vi "apply tracking setting.vi"(7 "tracking?":bool, 9 "tracking settings":T3, 10 "tracking state in":T1) -> (2 "tracking state out":T1={"x state"={"pos estimate"=0.0, "v estimate"=0.0, "weighted position error sum"=0.0, "photon count"=0, "transmit tick count"=0, "axis number"=0, "px (levels^2)"=0.0, "pxv (levels^2/ticks)"=0.0, "pv (levels^2/ticks^2)"=0.0, "vel diff (levels^2/ticks^3)"=0.0, "gx"=0.0, "rtwiddle"=0.0, "photon count ch0"=0, "photon count ch1"=0, "Dx -levels^2/ticks"=0.0}, "y state"={"pos estimate"=0.0, "v estimate"=0.0, "weighted position error sum"=0.0, "photon count"=0, "transmit tick count"=0, "axis number"=1, "px (levels^2)"=0.0, "pxv (levels^2/ticks)"=0.0, "pv (levels^2/ticks^2)"=0.0, "vel diff (levels^2/ticks^3)"=0.0, "gx"=0.0, "rtwiddle"=0.0, "photon count ch0"=0, "photon count ch1"=0, "Dx -levels^2/ticks"=0.0}, "z state"={"pos estimate"=0.0, "v estimate"=0.0, "weighted position error sum"=0.0, "photon count"=0, "transmit tick count"=0, "axis number"=2, "px (levels^2)"=0.0, "pxv (levels^2/ticks)"=0.0, "pv (levels^2/ticks^2)"=0.0, "vel diff (levels^2/ticks^3)"=0.0, "gx"=0.0, "rtwiddle"=0.0, "photon count ch0"=0, "photon count ch1"=0, "Dx -levels^2/ticks"=0.0}, "spot number"=0})   [LabVIEW 2010]
uses:
  polar tracking settings.ctl
  kalman 3-axis state.ctl
  integrating single axis kalman state.ctl
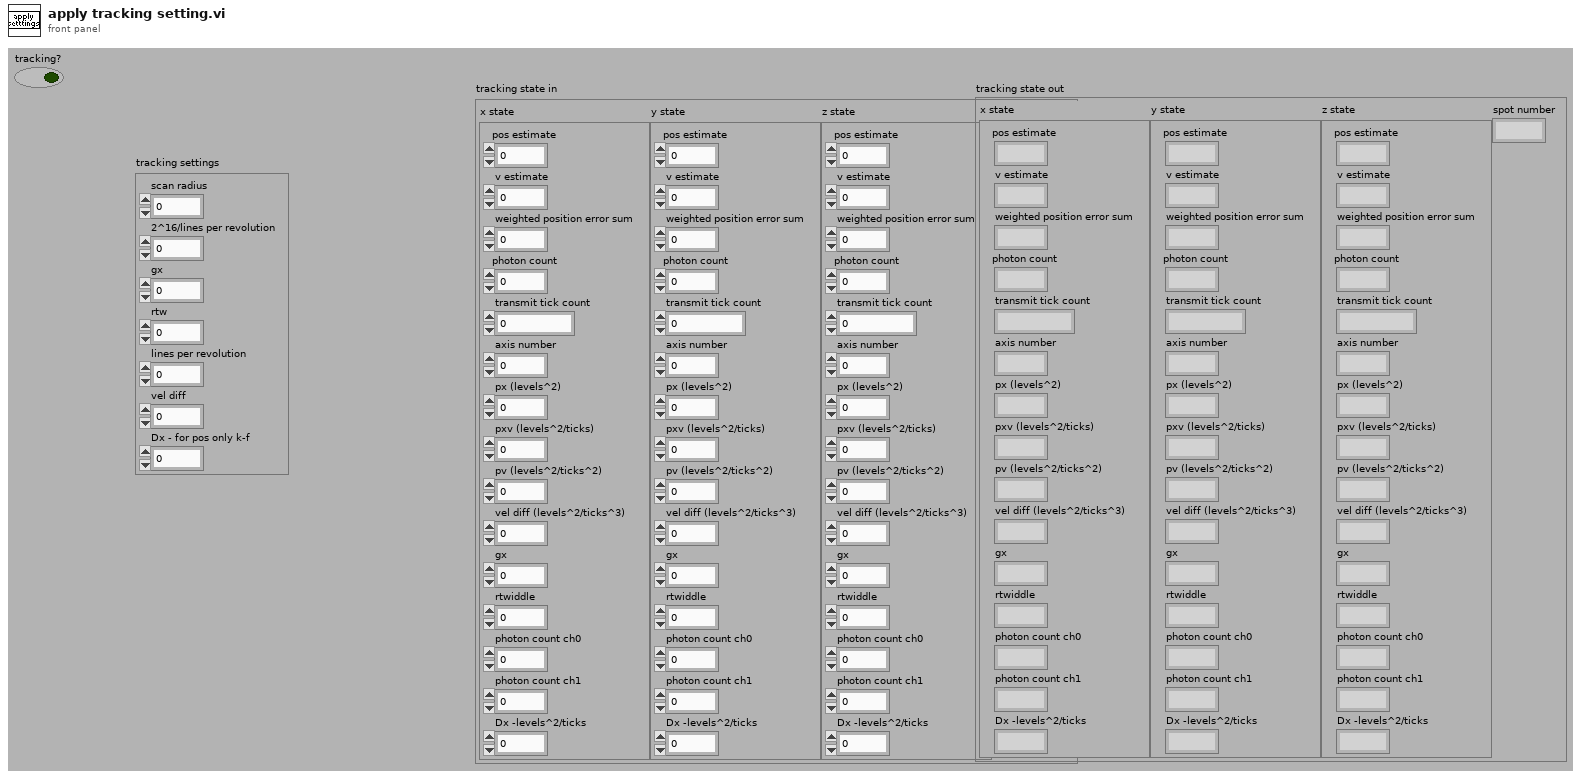
[diagram p1: front panel]
types:
  T1 = typedef "kalman 3-axis state.ctl" = cluster{"x state":T2, "y state":T2, "z state":T2, "spot number":u8}
  T2 = typedef "integrating single axis kalman state.ctl" = cluster{"pos estimate":fxp<+/-,32,16>, "v estimate":fxp<+/-,16,0>, "weighted position error sum":fxp<+/-,32,32>, "photon count":u32, "transmit tick count":u32, "axis number":u8, "px (levels^2)":fxp<+,32,19>, "pxv (levels^2/ticks)":fxp<+,32,2>, "pv (levels^2/ticks^2)":fxp<+,32,-14>, "vel diff (levels^2/ticks^3)":fxp<+,24,-22>, "gx":fxp<+,16,8>, "rtwiddle":fxp<+,16,26>, "photon count ch0":u32, "photon count ch1":u32, "Dx -levels^2/ticks":fxp<+,32,19>}
  T3 = typedef "polar tracking settings.ctl" = cluster{"scan radius":u16, "2^16/lines per revolution":u16, "gx":fxp<+,16,8>, "rtw":fxp<+,16,26>, "lines per revolution":u8, "vel diff":fxp<+,24,-22>, "Dx - for pos only k-f":fxp<+,32,19>}
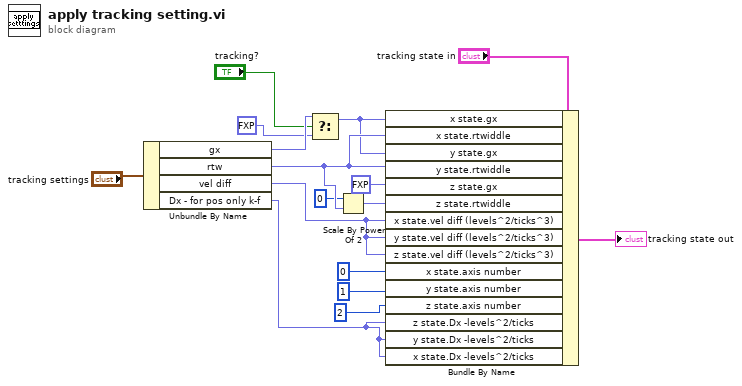
[diagram p0: block diagram]
diagram:
  n1 = Unbundle By Name("tracking settings") -> ("gx"=w3:fxp<+,16,8>, "rtw"=w13:fxp<+,16,26>, "vel diff"=w10:fxp<+,24,-22>, "Dx - for pos only k-f"=w6:fxp<+,32,19>)
  n2 = Select(t=w3, s="tracking?", f=fxp<+,16,8> 1.0) -> (s? t:f=w4:fxp<+,16,8>)
  n3 = Scale By Power Of 2(n=0, x=w13) -> (x*2^n=w11:fxp<+,16,26>)
  n4 = Bundle By Name(cluster="tracking state in", "x state.gx"=w4, "x state.rtwiddle"=w13, "y state.gx"=w4, "y state.rtwiddle"=w13, "z state.gx"=fxp<+,16,8> 1.0, "z state.rtwiddle"=w11, "x state.vel diff (levels^2/ticks^3)"=w10, "y state.vel diff (levels^2/ticks^3)"=w10, "z state.vel diff (levels^2/ticks^3)"=w10, "x state.axis number"=u8 0 ("x state.axes number"), "y state.axis number"=u8 1 ("y state.axes number"), "z state.axis number"=u8 2 ("z state.axes number"), "z state.Dx -levels^2/ticks"=w6, "y state.Dx -levels^2/ticks"=w6, "x state.Dx -levels^2/ticks"=w6) -> (→"tracking state out":T1)
